vi "Week 2 Digital Output.vi"() -> ()   [LabVIEW 2022 SP3]
uses:
  <vilib>/DAQmx/create/channels.llb/DAQmx Create Channel (DO-Digital Output).vi
  <vilib>/DAQmx/miscellaneous.llb/DAQmx Fill In Error Info.vi
panel:
  in  "data":bool
  out "Boolean":bool
  in  "stop":bool
  in  "lines":tag
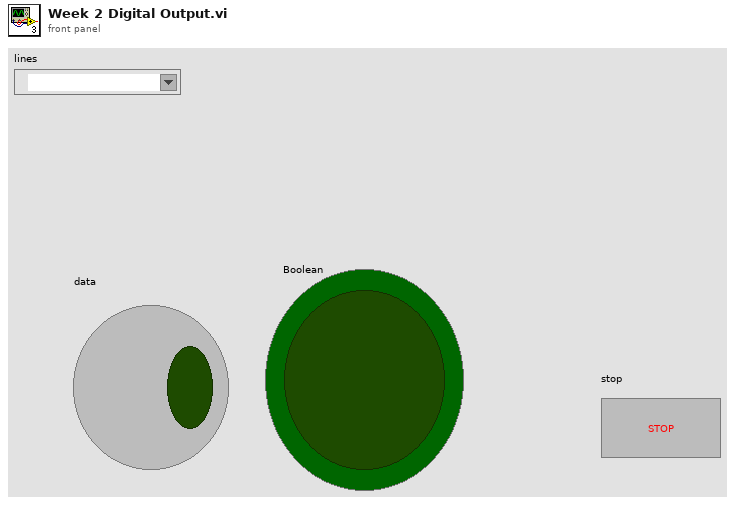
[diagram p1: front panel]
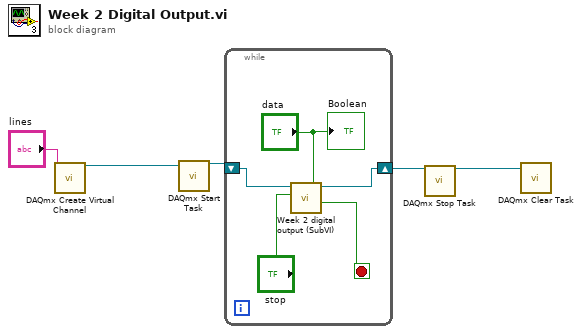
[diagram p0: block diagram]
diagram:
  n1 = call-poly <vilib>:"DAQmx Create Virtual Channel.vi"("lines"="lines") -> ("task out"=w4:refnum<k21>)  [unwired: 13 in, 1 out]
  n2 = call <vilib>:"DAQmx Start Task.vi"("task/channels in"=w4) -> ("task out"=w3:refnum<k21>)  [unwired: 13 in, 1 out]
  n3 = while {
    shift-right: [w9] -> w2
    shift-left: w3 -> [w10]
    stop <- w8 stop-if-true
    n4 = call "Week 2 digital output (SubVI).vi"("data"="data", "stop in"="stop", "Refnum in"=w10) -> ("stop out"=w8:bool, "Refnum out"=w9:refnum<k21>)  [unwired: 7 in]
    "Boolean" <- "data"
  }
  n5 = call <vilib>:"DAQmx Stop Task.vi"("task/channels in"=w2) -> ("task out"=w1:refnum<k21>)  [unwired: 13 in, 1 out]
  n6 = call <vilib>:"DAQmx Clear Task.vi"("task in"=w1) -> ()  [unwired: 14 in, 1 out]
